vi "set id.vi"(8 "error in (no error)":errorcluster, 10 "id":i32, 11 "img in":refnum<class "img.lvclass">) -> (0 "error out":errorcluster, 3 "img out":refnum<class "img.lvclass">)   [LabVIEW 2013, in "DatenKlassen.lvlib" / "img.lvclass"]
uses:
  img.lvclass
  img.lvclass/img.ctl
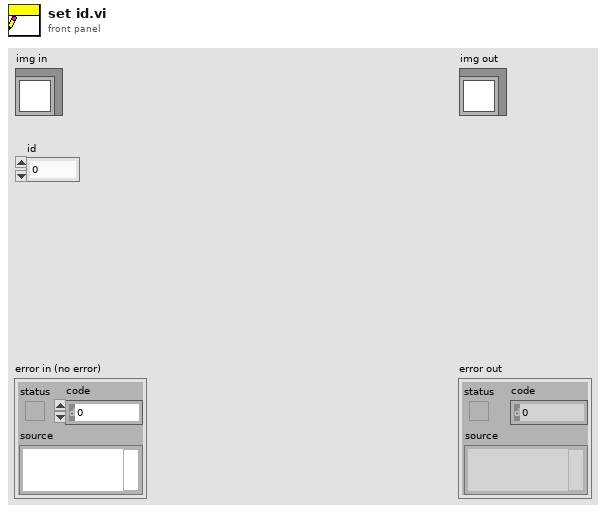
[diagram p1: front panel]
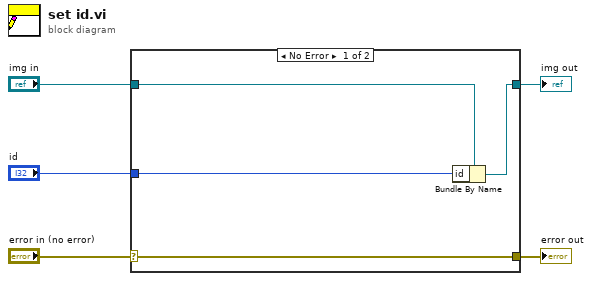
[diagram p0: block diagram]
diagram:
  n1 = case shown="No Error" "error in (no error)" {
    selector: "error in (no error)" -> [w9 w10]
    tunnel: [w9 w10] -> w4
    tunnel: [w7 w11] -> w2
    tunnel: "img in" -> [w8 w11]
    tunnel: "id" -> [w6 _]
    frame No Error {
      n2 = Bundle By Name(cluster=w8, "id"=w6) -> (w7:refnum<class "img.lvclass">)
    }
    frame Error {
    }
  }
  "error out" <- w4
  "img out" <- w2
